vi "Send Automation Event.vi"(8 "error in":errorcluster, 10 "Automation Reference":variant, 11 "Engine in":refnum<class "Engine.lvclass">) -> (0 "error out":errorcluster, 3 "Engine out":refnum<class "Engine.lvclass">)   [LabVIEW 2019, in "Engine.lvlib" / "Engine.lvclass"]
doc: "This allows TestStand to send a calling sequence reference in to the software. Ultimately, this allows any faults generated by the software to report up to TestStand to halt/abort testing."
uses:
  Project/Engine.lvclass
  Project/Engine.lvclass/Engine.ctl
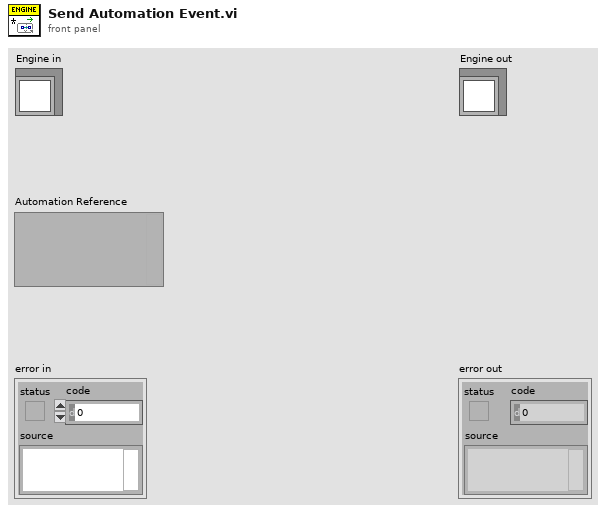
[diagram p1: front panel]
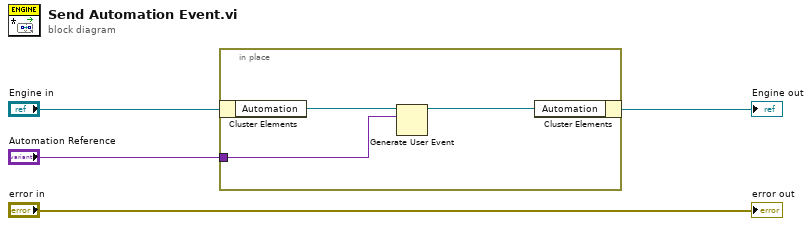
[diagram p0: block diagram]
diagram:
  n1 = in-place {
    in-place-border: "Automation Reference" -> [w5]
    n2 = in-place-cluster #1("Engine in") -> ("Automation"=w7:refnum<user-event>)
    n3 = Generate User Event(user event=w7, event data cluster=w5) -> (user event out=w6:refnum<user-event>)  [unwired: 2 in, 1 out]
    n4 = in-place-cluster #1("Automation"=w6) -> (→"Engine out":refnum<class "Engine.lvclass">)
  }
  "error out" <- "error in"
